vi "IsEnabled.vi"(8 "error in (no error)":errorcluster, 11 "reference in":refnum<class "DUT_Handler_Simple.lvclass">) -> (0 "error out":errorcluster, 1 "Enabled":bool, 3 "reference in":refnum<class "DUT_Handler_Simple.lvclass">)   [LabVIEW 2022 SP3, in "DUT_Handler_Simple.lvlib" / "DUT_Handler_Simple.lvclass"]
uses:
  DUT_Handler_Simple.lvclass
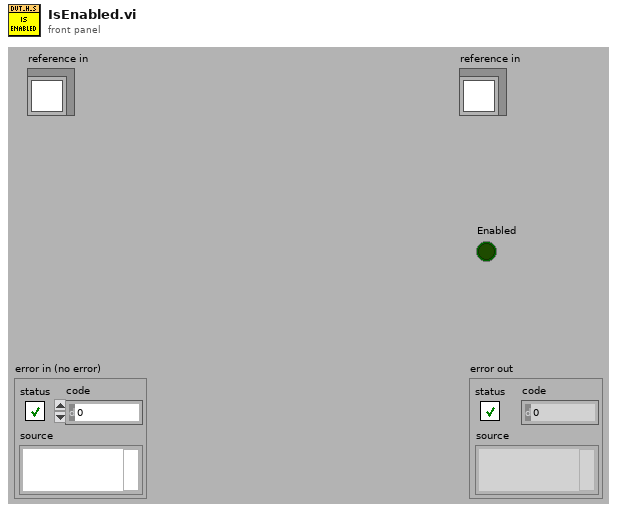
[diagram p1: front panel]
types:
  T1 = typedef "DUT_Handler_Simple.lvlib/DUT_Handler_Simple.lvclass/ObjectAttributes.ctl" = cluster{"Config":T2, "event_data":T3, "Enabled":bool, "Barcode_Reader":refnum<class "Barcode_Reader_Base.lvclass">}
  T2 = typedef "DUT_Handler_Simple.lvlib/DUT_Handler_Simple.lvclass/Config.ctl" = cluster{"default":string}
  T3 = typedef "DUT_Handler_Base.lvlibp/DUT_Handler_Base.lvclass/EventData.ctl" = cluster{"Action":enum16{"Load", "Cancel", "MoveIn", "MoveOut", "Abort", "Msg", "Enabled", "Disabled", "Fault", "Shutdown"}, "SN":string, "BN":string, "DUT__ID":u32, "Message":string, "From":string, "To":string}
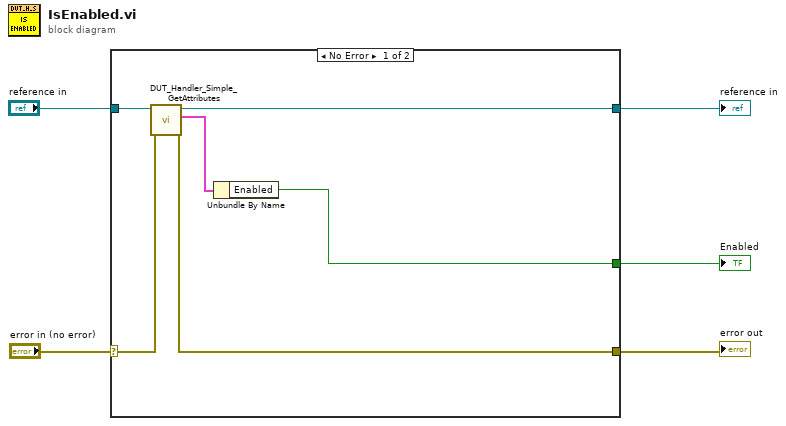
[diagram p0: block diagram]
diagram:
  n1 = case shown="No Error" "error in (no error)" {
    selector: "error in (no error)" -> [w11 w13]
    tunnel: [w9 w13] -> w4
    tunnel: [w7 w12] -> w2
    tunnel: "reference in" -> [w8 w12]
    tunnel: [w6 _] -> w1
    frame No Error {
      n2 = call "DUT_Handler_Simple_GetAttributes.vi"("error in (no error)"=w11, "reference in"=w8) -> ("error out"=w9:errorcluster, "Data"=w10:T1, "reference out"=w7:refnum<class "DUT_Handler_Simple.lvclass">)  [unwired: 6 in, 1 out]
      n3 = Unbundle By Name(w10) -> ("Enabled"=w6:bool)
    }
    frame Error {
    }
  }
  "error out" <- w4
  "reference in" <- w2
  "Enabled" <- w1
